vi "ZLIB Close Read File__ogtk.vi"(8 "error in (no error)":errorcluster, 9 "file timestamp (no change)":u32 format="%<%X\n%x>T", 10 "target path":path, 11 "unzip Refnum":T1) -> (0 "error out":errorcluster, 3 "unzip Refnum out":T1)   [LabVIEW 2014, in "ZLIB.lvlib"]
doc: "Closes a file opened with ZLIB Open Read File."
uses:
  ZLIB.lvlib
  ZLIB Unzip Handle__ogtk.ctl
  lvzlib.dll
panel:
  # "Please visit http://www.OpenG.org to learn about the\nOpen Source LabVIEW software movement.\n\nNOTICE -- YOU MUST LEAVE THIS NOTICE IN PLACE.  PER THE TERMS OF THE LICENSE BELOW, YOU MAY SUBLICENSE THIS SOFTWARE \nIN ANY WAY THAT DOES NOT CONFLICT WITH THIS LICENSE.\n\n### BSD License (http://www.opensource.org/licenses/bsd-license.php) Begin ###\n \nCopyright (C) 2002-2004 Rolf Kalbermatter rolf.kalbermatter@citeng.com\nCopyright (C) 2002 Jim Kring jim@jimkring.com\n\nAll rights reserved.\n\nRedistribution and use in source and binary forms, with or without modification, are permitted provided that the following conditions are met:\n\n    * Redistributions of source code must retain the above copyright notice, this list of conditions and the following disclaimer.\n    * Redistributions in binary form must reproduce the above copyright notice, this list of conditions and the following disclaimer in the \n       documentation and/or other materials provided with the distribution.\n    * Neither the name of SciWare, James Kring, Inc., nor the names of its contributors may be used to endorse or promote products derived \n       from this software without specific prior written permission.\n\nTHIS SOFTWARE IS PROVIDED BY THE COPYRIGHT HOLDERS AND CONTRIBUTORS \"AS IS\" AND ANY EXPRESS OR IMPLIED WARRANTIES, \nINCLUDING, BUT NOT LIMITED TO, THE IMPLIED WARRANTIES OF MERCHANTABILITY AND FITNESS FOR A PARTICULAR PURPOSE ARE \nDISCLAIMED. IN NO EVENT SHALL THE COPYRIGHT OWNER OR CONTRIBUTORS BE LIABLE FOR ANY DIRECT, INDIRECT, INCIDENTAL,\n SPECIAL, EXEMPLARY, OR CONSEQUENTIAL DAMAGES (INCLUDING, BUT NOT LIMITED TO, PROCUREMENT OF SUBSTITUTE GOODS OR \nSERVICES; LOSS OF USE, DATA, OR PROFITS; OR BUSINESS INTERRUPTION) HOWEVER CAUSED AND ON ANY THEORY OF LIABILITY, \nWHETHER IN CONTRACT, STRICT LIABILITY, OR TORT (INCLUDING NEGLIGENCE OR OTHERWISE) ARISING IN ANY WAY OUT OF THE USE \nOF THIS SOFTWARE, EVEN IF ADVISED OF THE POSSIBILITY OF SUCH DAMAGE.\n\n### BSD License End ###"
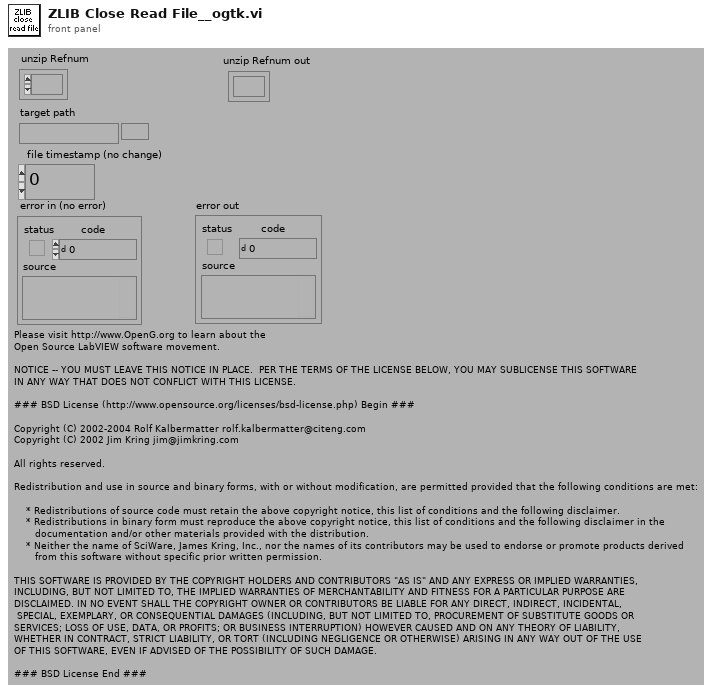
[diagram p1: front panel]
types:
  T1 = typedef "ZLIB.lvlib/ZLIB Unzip Handle__ogtk.ctl" = refnum<k1>
  T2 = typedef "ZLIB.lvlib/File Info Record__ogtk.ctl" = cluster{"type":string, "creator":string, "permissions":i32, "data size":i32, "res size":i32, "creation date":u32, "modification date":u32, "bFolder":bool, "bInvisible":bool, "location":cluster{"vertical":i16, "horizontal":i16}, "owner":string, "group":string}
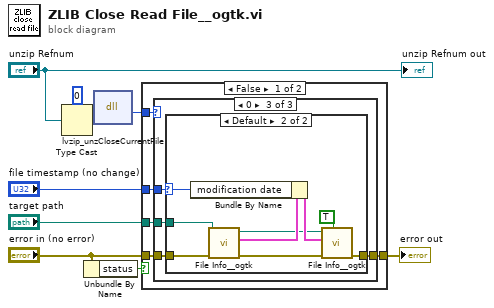
[diagram p0: block diagram]
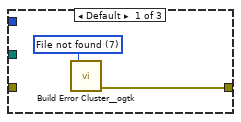
[diagram p2: hidden frame]
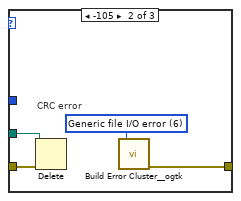
[diagram p3: hidden frame]
diagram:
  n1 = Type Cast(type=u32 0 ("unzFile"), x="unzip Refnum") -> (*(type *) &x=w6:u32)
  n2 = Unbundle By Name("error in (no error)") -> ("status"=w8:bool)
  n3 = dll-call lib="C:/Users/Public/SSDC/OpenDocument/LabVIEWODFToolkit/Sourcecode/SubVIs/ZLIB/lvzlib.*" fn="lvzip_unzCloseCurrentFile"("unzFile"=w6) -> (w4:i32)  [unwired: 4 in, 2 out]
  n4 = case shown="False" w8 {
    tunnel: "error in (no error)" -> [w14 w35]
    tunnel: [w13 w35] -> w9
    tunnel: w4 -> [w12 _]
    tunnel: "target path" -> [w11 _]
    tunnel: "file timestamp (no change)" -> [w10 _]
    frame False {
      n5 = case shown="0" w12 {
        tunnel: w14 -> [_ w17 w23]
        tunnel: [w16 w20 w22] -> w13
        tunnel: w11 -> [_ w18 w24]
        tunnel: w10 -> [_ _ w21]
        frame Default {
          w15 = 7 items=["No error", "Argument error", "Memory is full", "Out of zone", "End of file", "File already open", "Generic file I/O error", "File not found", "File permission error", "Disk is full", "Duplicate path", "Too many files open", "System feature not enabled", "Resource file not found", "Cannot add resource", "Resource not found", "Image not found", "Image memory error", "Pen does not exist", "Config type invalid", "Config token not found", "Config parse error", "Config memory error", "Bad external code format", "Bad external code offset", "External code not present", "Null window", "Destroy window error", "Null menu", "Print aborted", "Bad print record", "Print driver error", "Windows error during printing", "Memory error during printing", "Print dialog error", "Generic print error", "Invalid device refnum", "Device not found", "Device parameter error", "Device unit error", "Cannot open device", "Device call aborted", "Generic error", "Cancelled by user", "Object ID too low", "Object ID too high", "Object not in heap", "Unknown heap", "Unknown object (invalid DefProc)", "Unknown object (DefProc not in table)", "Message out of range", "Invalid (null) method", "Unknown message", "Manager call not supported", "Bad address", "Network operation in progress", "Network operation timed out", "Connection is busy", "Network attribute not supported", "Network error", "Address in use", "System out of memory", "Connection aborted", "Connection refused", "Not connected", "Already connected", "Connection closed", "Initialization error (interapplication manager)", "Bad occurrence", "Wait on unbound occurrence handler", "Occurrence queue overflow", "Datalog type conflict", "Unused", "Unrecognized type (interapplication manager)", "Memory corrupt", "Failed to make temporary DLL", "Old CIN version", "Drag socket not found", "Failed to load drop-object", "Failed to register OLE object", "Failed to release OLE object", "Format specifier type mismatch", "Unknown format specifier", "Too few format specifiers", "Too many format specifiers", "Scan failed", "Newer CIN version", "Error converting to variant", "Runtime menu error", "Password tampered", "Variant attribute not found", "Incompatible variant data type", "Event data is not available", "Event Store is not present", "Occurrence is not found", "Event Queue is not created", "Event info is not available", "Refnum passed is NULL", "Error retrieving Class GUID", "Error retrieving CoClass GUID", "Error retrieving TypeLib GUID.", "Bad built application magic bytes.", "Specific driver is different from the specific driver associated with the Logical Name.", "There is no session opened to the class driver.", "Max Error", "MAX - Error with config objects", "MAX - Error loading configuration", "MAX - Group not supported"]
          n6 = call "Build Error Cluster__ogtk.vi"("code"=w15) -> ("error out"=w16:errorcluster)  [unwired: 1 in]
        }
        frame -105 {
          w19 = 6 items=["No error", "Argument error", "Memory is full", "Out of zone", "End of file", "File already open", "Generic file I/O error", "File not found", "File permission error", "Disk is full", "Duplicate path", "Too many files open", "System feature not enabled", "Resource file not found", "Cannot add resource", "Resource not found", "Image not found", "Image memory error", "Pen does not exist", "Config type invalid", "Config token not found", "Config parse error", "Config memory error", "Bad external code format", "Bad external code offset", "External code not present", "Null window", "Destroy window error", "Null menu", "Print aborted", "Bad print record", "Print driver error", "Windows error during printing", "Memory error during printing", "Print dialog error", "Generic print error", "Invalid device refnum", "Device not found", "Device parameter error", "Device unit error", "Cannot open device", "Device call aborted", "Generic error", "Cancelled by user", "Object ID too low", "Object ID too high", "Object not in heap", "Unknown heap", "Unknown object (invalid DefProc)", "Unknown object (DefProc not in table)", "Message out of range", "Invalid (null) method", "Unknown message", "Manager call not supported", "Bad address", "Network operation in progress", "Network operation timed out", "Connection is busy", "Network attribute not supported", "Network error", "Address in use", "System out of memory", "Connection aborted", "Connection refused", "Not connected", "Already connected", "Connection closed", "Initialization error (interapplication manager)", "Bad occurrence", "Wait on unbound occurrence handler", "Occurrence queue overflow", "Datalog type conflict", "Unused", "Unrecognized type (interapplication manager)", "Memory corrupt", "Failed to make temporary DLL", "Old CIN version", "Drag socket not found", "Failed to load drop-object", "Failed to register OLE object", "Failed to release OLE object", "Format specifier type mismatch", "Unknown format specifier", "Too few format specifiers", "Too many format specifiers", "Scan failed", "Newer CIN version", "Error converting to variant", "Runtime menu error", "Password tampered", "Variant attribute not found", "Incompatible variant data type", "Event data is not available", "Event Store is not present", "Occurrence is not found", "Event Queue is not created", "Event info is not available", "Refnum passed is NULL", "Error retrieving Class GUID", "Error retrieving CoClass GUID", "Error retrieving TypeLib GUID.", "Bad built application magic bytes.", "Specific driver is different from the specific driver associated with the Logical Name.", "There is no session opened to the class driver.", "Max Error", "MAX - Error with config objects", "MAX - Error loading configuration", "MAX - Group not supported"]
          # "CRC error"
          n7 = Delete(path (use dialog)=w18, error in=w17) -> ()  [unwired: 3 in, 3 out]
          n8 = call "Build Error Cluster__ogtk.vi"("code"=w19) -> ("error out"=w20:errorcluster)  [unwired: 1 in]
        }
        frame 0 {
          n9 = case shown="Default" w21 {
            selector: w21 -> [_ w26]
            tunnel: w23 -> [w25 w33]
            tunnel: w24 -> [_ w34]
            tunnel: [w25 w27] -> w22
            frame 0 {
            }
            frame Default {
              n10 = call "File Info__ogtk.vi"("error in (no error)"=w33, "file"=w34) -> ("error out"=w32:errorcluster, "file info"=w31:T2, "file out"=w29:path)  [unwired: 4 in]
              n11 = Bundle By Name(cluster=w31, "modification date"=w26) -> (w30:T2)
              n12 = call "File Info__ogtk.vi"("update (F)"=TRUE ("write (F)"), "error in (no error)"=w32, "file info"=w30, "file"=w29) -> ("error out"=w27:errorcluster)  [unwired: 2 in, 2 out]
            }
          }
        }
      }
    }
    frame True {
    }
  }
  "error out" <- w9
  "unzip Refnum out" <- "unzip Refnum"
